vi "ArrayGlobal_radial.vi"(0 "Function":T1(ring), 1 "Galga2":dbl[](array[numeric]) format="%.2f", 2 "Galga1":dbl[](array[numeric]) format="%.2f", 3 "Galga3":dbl[](array[numeric]) format="%.2f", 4 "Galga4":dbl[](array[numeric]) format="%.2f", 5 "Promedio":dbl[](array[numeric]) format="%.2f", 6 "Path":path, 9 "Bomba":dbl[](array[numeric]) format="%.2f", 11 "Tiempo":dbl[](array[numeric]) format="%.2f") -> (16 "ArrayOut":dbl[](array[numeric]) format="%.2f")   [LabVIEW 2015]
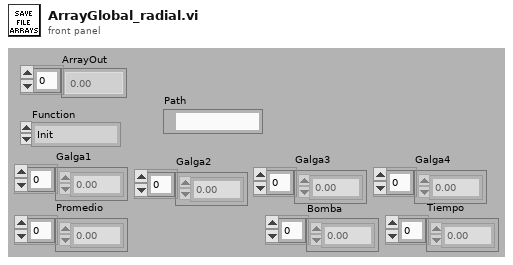
[diagram p1: front panel]
types:
  T1 = enum16{"Init", "Write", "Read array", "Read subarray"}
  T2 = enum16{"open", "open or create", "create or replace", "create", "open (read-only)"}
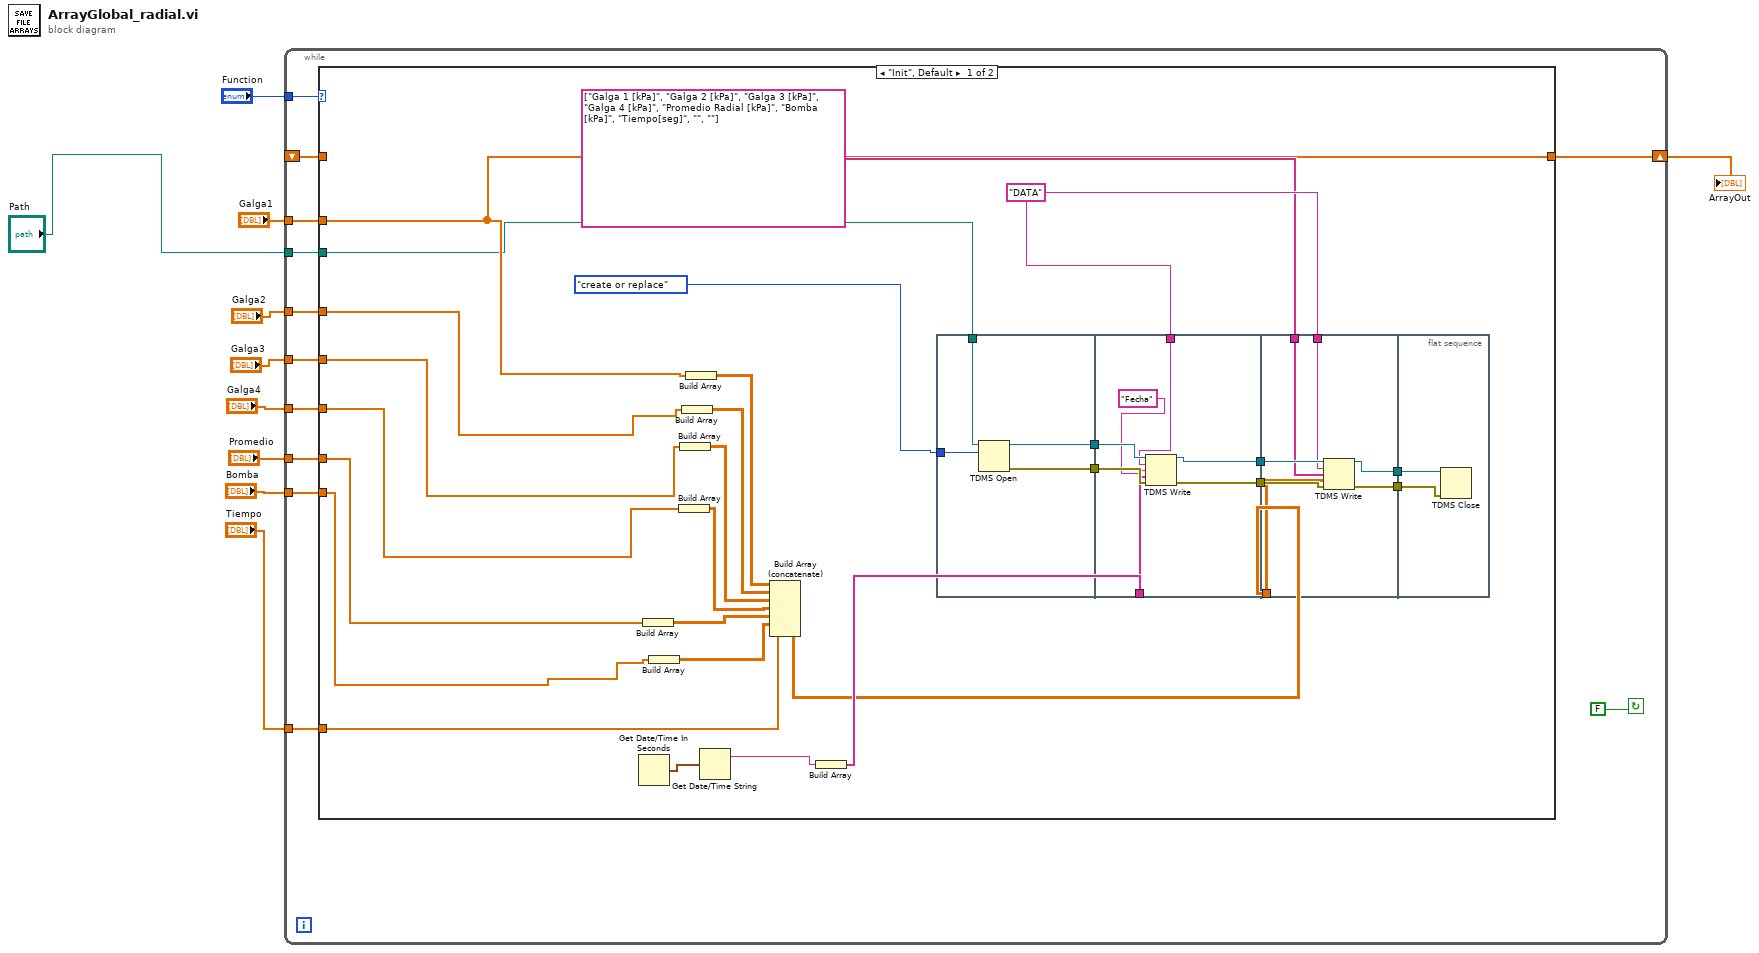
[diagram p0: block diagram]
diagram:
  n1 = while {
    tunnel: "Function" -> [w22]
    shift-right: [w21] -> w8
    shift-left: _ -> [w20]
    tunnel: "Galga1" -> [w19]
    tunnel: "Galga2" -> [w17]
    tunnel: "Galga3" -> [w16]
    tunnel: "Galga4" -> [w15]
    tunnel: "Promedio" -> [w14]
    tunnel: "Bomba" -> [w13]
    tunnel: "Tiempo" -> [w12]
    tunnel: "Path" -> [w11]
    stop <- FALSE continue-if-true
    n2 = case shown="\"Init\", Default" w22 {
      tunnel: [w25 w70] -> w21
      tunnel: w20 -> [_ w70]
      tunnel: w19 -> [w25 _]
      tunnel: w17 -> [w30 _]
      tunnel: w16 -> [w29 _]
      tunnel: w15 -> [w28 _]
      tunnel: w14 -> [w27 _]
      tunnel: w13 -> [w26 _]
      tunnel: w12 -> [w24 _]
      tunnel: w11 -> [w23 _]
      frame "Init", Default {
        w35 = "DATA"
        n3 = Get Date/Time In Seconds() -> (seconds since 1Jan1904=w37:timestamp)
        n4 = Build Array(w27) -> (w39:dbl[][])
        n5 = Build Array(w26) -> (w38:dbl[][])
        n6 = Build Array(w28) -> (w43:dbl[][])
        n7 = Build Array(w29) -> (w40:dbl[][])
        n8 = Build Array(w30) -> (w41:dbl[][])
        n9 = Build Array(w25) -> (w42:dbl[][])
        n10 = Get Date/Time String(seconds (now)=w37) -> (date string=w31:string)  [unwired: 2 in, 1 out]
        n11 = Build Array (concatenate)(w42, w41, w40, w43, w39, w38, w24) -> (w33:dbl[][])
        n12 = Build Array(w31) -> (w36:string[])
        n13 = flat-sequence {
          tunnel: T2."create or replace" ("operation (0:open)") -> [w53]
          tunnel: w23 -> [w52]
          tunnel: [w51] -> w49
          tunnel: [w50] -> w48
          tunnel: w49 -> [w60]
          tunnel: w48 -> [w59]
          tunnel: [w58] -> w47
          tunnel: [w57] -> w46
          tunnel: w35 -> [w55]
          tunnel: w36 -> [w54]
          tunnel: w47 -> [w67]
          tunnel: [w66] -> w45
          tunnel: [w65] -> w44
          tunnel: w46 -> [w64]
          tunnel: w35 -> [w63]
          tunnel: string[] ["Galga 1 [kPa]", "Galga 2 [kPa]", "Galga 3 [kPa]", "Galga 4 [kPa]", "Promedio Radial [kPa]", "Bomba [kPa]", "Tiempo[seg]", "", ""] ("channel name(s) in (Untitled)") -> [w62]
          tunnel: w33 -> [w61]
          tunnel: w45 -> [w69]
          tunnel: w44 -> [w68]
          frame #0 {
            n14 = TDMS Open(10:w53, 11:w52) -> (0:w50:errorcluster, 3:w51:refnum<k34>)  [unwired: 5 in]
          }
          frame #1 {
            n15 = TDMS Write(0:w60, 5:w55, 7:"Fecha" ("channel name(s) in (Untitled)"), 9:w54, 11:w59) -> (4:w58:refnum<k34>, 15:w57:errorcluster)  [unwired: 1 in, 2 out]
          }
          frame #2 {
            n16 = TDMS Write(0:w67, 5:w63, 7:w62, 9:w61, 11:w64) -> (4:w66:refnum<k34>, 15:w65:errorcluster)  [unwired: 1 in, 2 out]
          }
          frame #3 {
            n17 = TDMS Close(8:w68, 11:w69) -> ()  [unwired: 2 out]
          }
        }
      }
      frame "Read array" {
      }
    }
  }
  "ArrayOut" <- w8
